vi "IS Send One-shot.vi"(6 "Stream Time (optional)":timestamp=timestamp(1451714400 s since 1904-01-01), 7 "Access Key":string, 8 "error in (no error)":errorcluster, 9 "Numeric":dbl, 10 "Stream Key":string, 11 "Bucket Key":string) -> (0 "error out":errorcluster, 1 "Rate Limit Reached?":bool)   [LabVIEW 2013]
doc: "This VI wraps an entire request into a single VI. You provide a valid Access Key and Bucket Key to send data to a specific place in Initial State. You then provide a simple data point (as a DBL), name the stream with a Stream Key, and optionally provide a timestamp. If you do not provide a timestamp, current Data/Time is passed through the API. This is the simplest way to stream any data from anywhere in your system with one VI."
uses:
  Data Helpers/IS PolyVI Instance DBL To JSON Cluster .vi
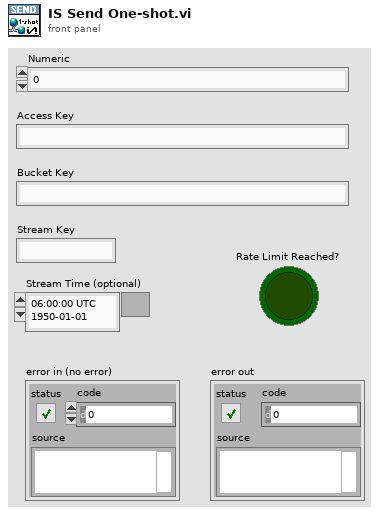
[diagram p1: front panel]
types:
  T1 = typedef "IS Session.ctl" = cluster{"Access Key":string, "HTTP Client Handle":T2}
  T2 = typedef "LabVIEWHTTPClient.lvlib/ClientHandle.ctl" = refnum<k1>
  T3 = typedef "IS Data Point TypeDef (String).ctl" = cluster{"key":string, "value":string, "epoch":dbl}
  T4 = typedef "IS Bucket Session.ctl" = cluster{"Bucket Key":string}
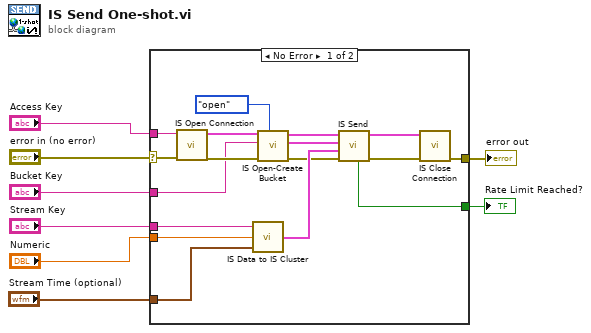
[diagram p0: block diagram]
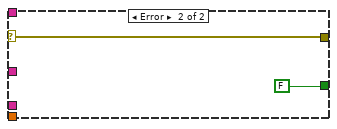
[diagram p2: hidden frame]
diagram:
  n1 = case shown="No Error" "error in (no error)" {
    selector: "error in (no error)" -> [w11 w27]
    tunnel: [w25 w27] -> w8
    tunnel: "Stream Key" -> [w21 _]
    tunnel: "Numeric" -> [w20 _]
    tunnel: "Bucket Key" -> [w15 _]
    tunnel: "Access Key" -> [w13 _]
    tunnel: "Stream Time (optional)" -> [w10 _]
    tunnel: [w9 FALSE] -> w1
    frame No Error {
      n2 = call "IS Open Connection.vi"("error in (no error)"=w11, "Access Key"=w13) -> ("error out"=w16:errorcluster, "IS Session"=w14:T1)  [unwired: 8 in]
      n3 = call-poly "IS Data to IS Cluster.vi"("Stream Time (optional)"=w10, "Stream Value"=w20, "Stream Key"=w21) -> ("JSON Cluster Array out"=w22:T3[])  [unwired: 2 in]
      n4 = call "IS Open-Create Bucket.vi"("Operation (0: open)"=enum16{"open", "create"}."open", "error in (no error)"=w16, "Bucket Key (Optional)"=w15, "IS Session In"=w14) -> ("error IO"=w17:errorcluster, "IS Bucket Session"=w19:T4, "IS Session Out"=w18:T1)  [unwired: 5 in]
      n5 = call "IS Send.vi"("error in (no error)"=w17, "JSON Custer Array in"=w22, "IS Bucket Session"=w19, "IS Session in"=w18) -> ("Error out"=w23:errorcluster, "IS Session out"=w24:T1, "Rate Limit Reached?"=w9:bool)  [unwired: 2 in, 3 out]
      n6 = call "IS Close Connection.vi"("error in (no error)"=w23, "IS Session In"=w24) -> ("error out"=w25:errorcluster)  [unwired: 9 in]
    }
    frame Error {
    }
  }
  "error out" <- w8
  "Rate Limit Reached?" <- w1
